vi "Configure Limit Test.vi"(8 "error in (no error)":errorcluster, 9 "Enable Limit Test (Disable)":bool, 10 "Measurement Type (6: Phase Noise)":u16(ring)=6 items=["AM Noise"=1, "Baseband Noise"=2, "Freq/Power"=3, "Spectrum"=4, "Transient"=5, "Phase Noise"=6, "User"=7], 11 "VISA resource name":refnum<visa-resource-name>) -> (0 "error out":errorcluster, 3 "VISA resource name out":refnum<visa-resource-name>)   [LabVIEW 2011, in "Agilent E5052X.lvlib"]
doc: "Configures limit testing for all measurements."
uses:
  Agilent E5052X.lvlib
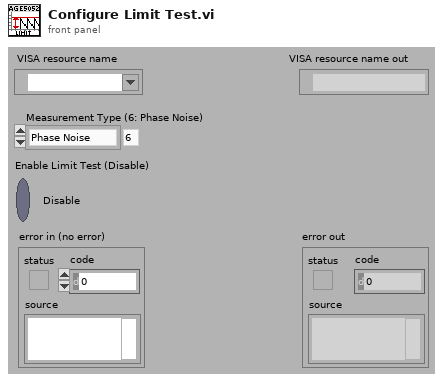
[diagram p1: front panel]
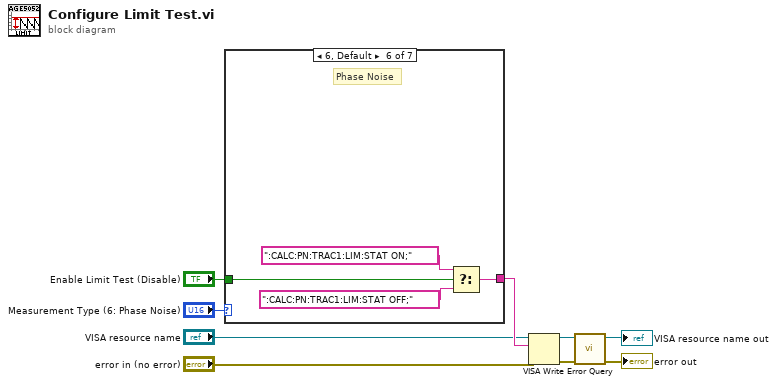
[diagram p0: block diagram]
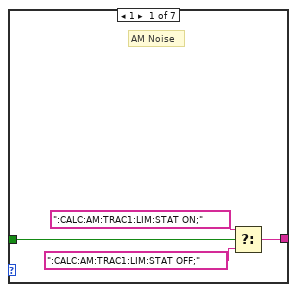
[diagram p2: hidden frame]
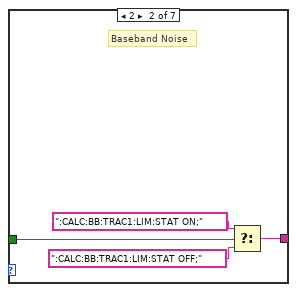
[diagram p3: hidden frame]
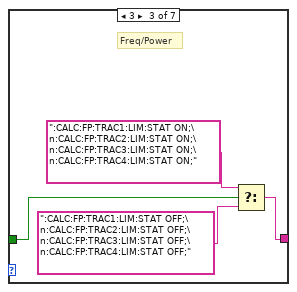
[diagram p4: hidden frame]
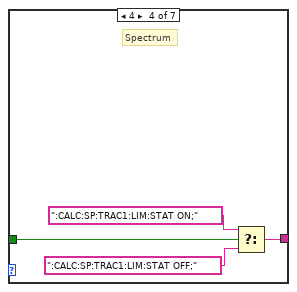
[diagram p5: hidden frame]
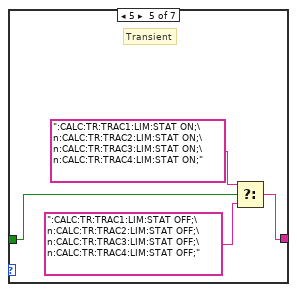
[diagram p6: hidden frame]
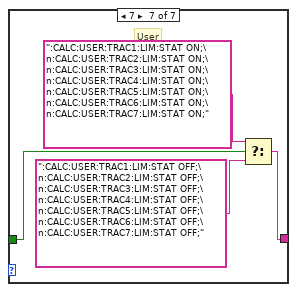
[diagram p7: hidden frame]
diagram:
  n1 = case shown="6, Default" "Measurement Type (6: Phase Noise)" {
    tunnel: "Enable Limit Test (Disable)" -> [w11 w15 w19 w23 w27 w30 w34]
    tunnel: [w10 w14 w18 w22 w26 w31 w35] -> w4
    frame 1 {
      # "AM Noise"
      n2 = Select(t=":CALC:AM:TRAC1:LIM:STAT ON;", s=w11, f=":CALC:AM:TRAC1:LIM:STAT OFF;") -> (s? t:f=w10:string)
    }
    frame 2 {
      # "Baseband Noise"
      n3 = Select(t=":CALC:BB:TRAC1:LIM:STAT ON;", s=w15, f=":CALC:BB:TRAC1:LIM:STAT OFF;") -> (s? t:f=w14:string)
    }
    frame 3 {
      # "Freq/Power"
      n4 = Select(t=":CALC:FP:TRAC1:LIM:STAT ON;\n:CALC:FP:TRAC2:LIM:STAT ON;\n:CALC:FP:TRAC3:LIM:STAT ON;\n:CALC:FP:TRAC4:LIM:STAT ON;", s=w19, f=":CALC:FP:TRAC1:LIM:STAT OFF;\n:CALC:FP:TRAC2:LIM:STAT OFF;\n:CALC:FP:TRAC3:LIM:STAT OFF;\n:CALC:FP:TRAC4:LIM:STAT OFF;") -> (s? t:f=w18:string)
    }
    frame 4 {
      # "Spectrum"
      n5 = Select(t=":CALC:SP:TRAC1:LIM:STAT ON;", s=w23, f=":CALC:SP:TRAC1:LIM:STAT OFF;") -> (s? t:f=w22:string)
    }
    frame 5 {
      # "Transient"
      n6 = Select(t=":CALC:TR:TRAC1:LIM:STAT ON;\n:CALC:TR:TRAC2:LIM:STAT ON;\n:CALC:TR:TRAC3:LIM:STAT ON;\n:CALC:TR:TRAC4:LIM:STAT ON;", s=w27, f=":CALC:TR:TRAC1:LIM:STAT OFF;\n:CALC:TR:TRAC2:LIM:STAT OFF;\n:CALC:TR:TRAC3:LIM:STAT OFF;\n:CALC:TR:TRAC4:LIM:STAT OFF;") -> (s? t:f=w26:string)
    }
    frame 6, Default {
      # "Phase Noise"
      n7 = Select(t=":CALC:PN:TRAC1:LIM:STAT ON;", s=w30, f=":CALC:PN:TRAC1:LIM:STAT OFF;") -> (s? t:f=w31:string)
    }
    frame 7 {
      # "User"
      n8 = Select(t=":CALC:USER:TRAC1:LIM:STAT ON;\n:CALC:USER:TRAC2:LIM:STAT ON;\n:CALC:USER:TRAC3:LIM:STAT ON;\n:CALC:USER:TRAC4:LIM:STAT ON;\n:CALC:USER:TRAC5:LIM:STAT ON;\n:CALC:USER:TRAC6:LIM:STAT ON;\n:CALC:USER:TRAC7:LIM:STAT ON;", s=w34, f=":CALC:USER:TRAC1:LIM:STAT OFF;\n:CALC:USER:TRAC2:LIM:STAT OFF;\n:CALC:USER:TRAC3:LIM:STAT OFF;\n:CALC:USER:TRAC4:LIM:STAT OFF;\n:CALC:USER:TRAC5:LIM:STAT OFF;\n:CALC:USER:TRAC6:LIM:STAT OFF;\n:CALC:USER:TRAC7:LIM:STAT OFF;") -> (s? t:f=w35:string)
    }
  }
  n9 = VISA Write(VISA resource name="VISA resource name", write buffer=w4, error in (no error)="error in (no error)") -> (VISA resource name out=w8:refnum<visa-resource-name>, error out=w7:errorcluster)  [unwired: 1 out]
  n10 = call "Error Query.vi"("error in (no error)"=w7, "VISA resource name"=w8) -> ("error out"=→"error out":errorcluster, "VISA resource name out"=→"VISA resource name out":refnum<visa-resource-name>)  [unwired: 6 in, 2 out]
